vi "DAQ_Task_Counter.vi"(8 "error in":errorcluster, 10 "Action":enum16{"Init", "Write", "Read"}(ring), 11 "DAQ_Task_Counter":refnum<k21>) -> (0 "error out":errorcluster, 3 "DAQ_Task_Counter":refnum<k21>)   [LabVIEW 2025]
doc: "Functional Global Variable:\n- Write the value into the memory \nor\n- Read the value from the memory"
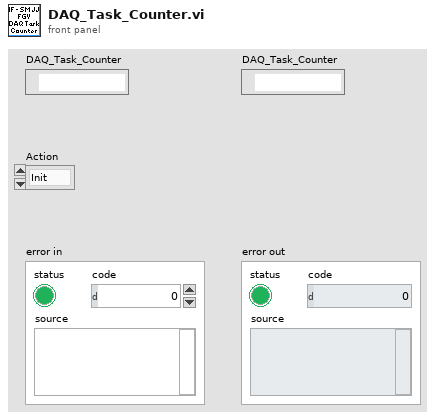
[diagram p1: front panel]
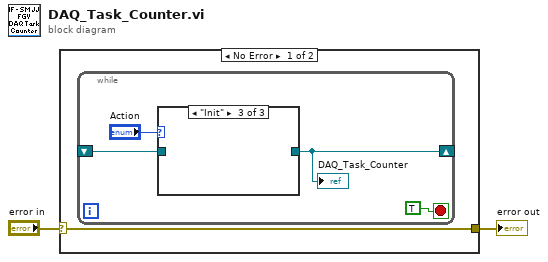
[diagram p0: block diagram]
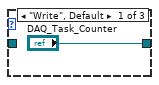
[diagram p2: hidden frame]
diagram:
  n1 = case shown="No Error" "error in" {
    selector: "error in" -> [w3 w10]
    tunnel: [w3 w10] -> w1
    frame No Error {
      n2 = while {
        shift-right: [w4] -> _
        shift-left: _ -> [w5]
        stop <- TRUE stop-if-true
        n3 = case shown="\"Init\"" "Action" {
          tunnel: w5 -> [_ w9 _]
          tunnel: ["DAQ_Task_Counter" w9 _] -> w4
          frame "Write", Default {
          }
          frame "Read" {
          }
          frame "Init" {
          }
        }
        "DAQ_Task_Counter" <- w4
      }
    }
    frame Error {
    }
  }
  "error out" <- w1
